vi "Example Threshold.vi"() -> ()   [LabVIEW 2010]
uses:
  C:/tf/play/labview/Tinkerforge.dll
  Tinkerforge.dll
panel:
  in  "stop":bool
  out "callback counter":i32
  out "last uvi":sgl
  in  "uid":string="amb"
  in  "port":i32=4223
  in  "host":string="localhost"
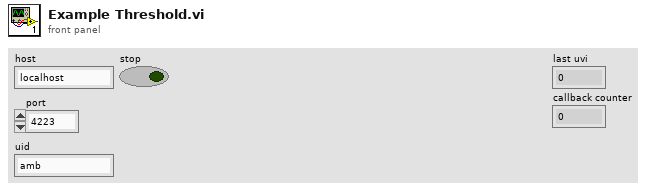
[diagram p1: front panel]
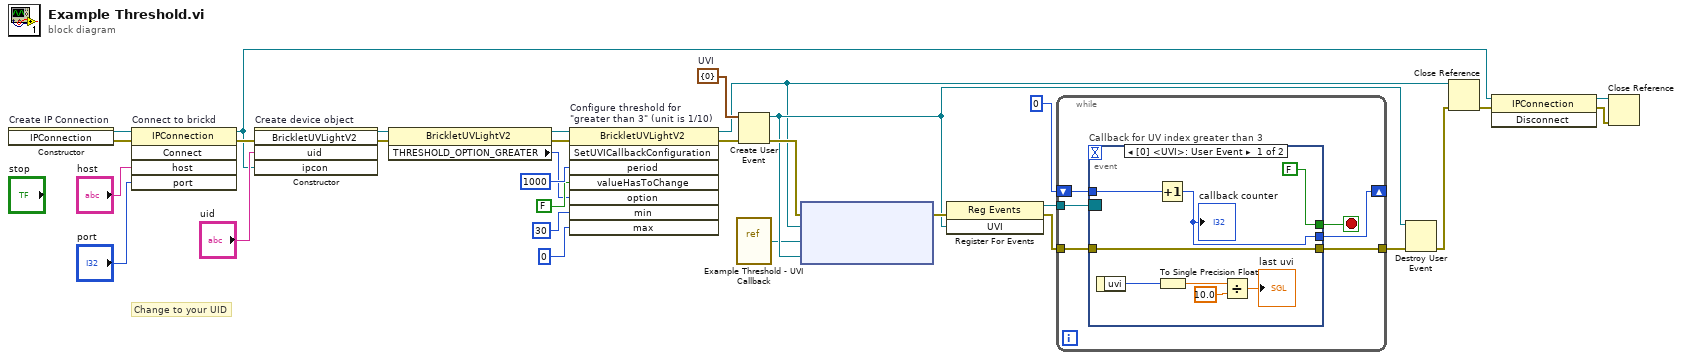
[diagram p0: block diagram]
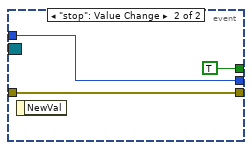
[diagram p2: hidden frame]
diagram:
  w15 = cluster{"uvi":i32} {"uvi"=0}  # UVI
  # "Change to your UID"
  n1 = constructor on="Create IP Connection" class="IPConnection"() -> (reference out=w31:refnum<k24>, error out=w9:errorcluster)  [unwired: 3 in, 1 out]
  n2 = invoke on="Connect to brickd" class="IPConnection" method="Connect"(reference=w31, error in=w9, "host"="host", "port"="port") -> (reference out=w24:refnum<k24>, error out=w27:errorcluster)  [unwired: 1 in, 3 out]
  n3 = constructor on="Create device object" class="BrickletUVLightV2"(error in=w27, "uid"="uid", "ipcon"=w24) -> (reference out=w2:refnum<k24>, error out=w1:errorcluster)  [unwired: 2 in, 3 out]
  n4 = property class="BrickletUVLightV2"(reference=w2, error in=w1) -> (reference out=w11:refnum<k24>, error out=w12:errorcluster, "THRESHOLD_OPTION_GREATER"=w6:u16)
  n5 = invoke on="Configure threshold for\n\"greater than 3\" (unit is 1/10)" class="BrickletUVLightV2" method="SetUVICallbackConfiguration"(reference=w11, error in=w12, "period"=i64 1000, "valueHasToChange"=FALSE, "option"=w6, "min"=30, "max"=0) -> (reference out=w14:refnum<k24>, error out=w13:errorcluster)  [unwired: 1 in, 6 out]
  n6 = vi-ref "Example Threshold - UVI Callback.vi"() -> ("vi reference"=w3:refnum<vi>)
  n7 = Create User Event(user event datatype=w15, error in=w13) -> (user event=w17:refnum<user-event>, error out=w22:errorcluster)
  n8 = node ("Register Event Callback")(w22, w14, w3, w17) -> (w21:errorcluster)  [unwired: 1 in, 1 out]
  n9 = register-events(error in=w21, w17) -> (reference out=w20:refnum<event-registration>, error out=w18:errorcluster)  [unwired: 1 in]
  n10 = while {
    tunnel: w20 -> [w37]
    tunnel: [w36] -> w19
    tunnel: w18 -> [w35]
    shift-right: [w33] -> _
    shift-left: 0 -> [w34]
    stop <- w32 stop-if-true
    n11 = event "Callback for UV index greater than 3" shown="[0] <UVI>: User Event" {
      selector: w37 -> [_ _]
      dyn-events: _ -> [_ _]
      timeout: _ -> [_ _]
      tunnel: [w42 w47] -> w36
      tunnel: w35 -> [w42 w47]
      tunnel: w34 -> [w40 w46]
      tunnel: [w39 w46] -> w33
      tunnel: [FALSE TRUE] -> w32
      event User Event {
        n12 = event-data() -> ("uvi"=w43:i32)  [unwired: 1 in]
        n13 = Increment(x=w40) -> (x+1=w39:i32)
        "callback counter" <- w39
        n14 = To Single Precision Float(number=w43) -> (single precision float=w44:sgl)
        n15 = Divide(x=w44, y=sgl 10.0) -> (x/y=→"last uvi":sgl)
      }
      event "stop": Value Change {
        n16 = event-data() -> ()  [unwired: 1 in, 1 out]
      }
    }
  }
  n17 = Destroy User Event(user event=w17, error in=w19) -> (error out=w16:errorcluster)
  n18 = Close Reference(reference=w14, error in (no error)=w16) -> (error out=w26:errorcluster)
  n19 = invoke class="IPConnection" method="Disconnect"(reference=w24, error in=w26) -> (reference out=w23:refnum<k24>, error out=w25:errorcluster)  [unwired: 1 in, 1 out]
  n20 = Close Reference(reference=w23, error in (no error)=w25) -> ()  [unwired: 1 out]
